vi "ZDataVIS_LineCuts.vi"(4 "Intensity Plot":refnum<vi>, 6 "e^2/h?":bool, 7 "tpose":bool, 8 "error in (no error)":errorcluster, 9 "Decimated X values":dbl[](array[numeric]), 10 "Arr of Y arrays (intensity info)":dbl[][](array[numeric]), 11 "State Wire IN":T1={"Core"={"Current VI Reference"=refnum, "Close Panel on Exit?"=FALSE}, "Sweep Data Cluster"={"Vfast"=[], "Vslow"=[], "Vslowest"=[], "Comments"="", "Scan names"=[]}, "Cursor Info"={"Fast Index"=[], "Slow Index"=0.0, "Slow Indices"=[], "Raw Cursor Position"={"X"=0.0, "Y"=0.0}, "Field / temp"=0}, "Scan names"=[], "Data DVR"=refnum, "Arr of Y arrays (intensity info)"=[], "Decimated X values"=[], "X Step Info"={"X Low"=-0.1, "X High"=0.1, "X Step"=4e-05}, "Voffset -2T"=0.0} {"X Step Info"."X Step" format="%#_6p"; "X Step Info"."X High" format="%#_6p"; "X Step Info"."X Low" format="%#_6p"}) -> (0 "error out":errorcluster, 1 "X line cut":cluster{dbl[], dbl[]}(graph), 2 "Y line cut":cluster{"Vfast":dbl[], dbl[]}(graph), 3 "State Wire OUT":T1={"Core"={"Current VI Reference"=refnum, "Close Panel on Exit?"=FALSE}, "Sweep Data Cluster"={"Vfast"=[], "Vslow"=[], "Vslowest"=[], "Comments"="", "Scan names"=[]}, "Cursor Info"={"Fast Index"=[], "Slow Index"=0.0, "Slow Indices"=[], "Raw Cursor Position"={"X"=0.0, "Y"=0.0}, "Field / temp"=0}, "Scan names"=[], "Data DVR"=refnum, "Arr of Y arrays (intensity info)"=[], "Decimated X values"=[], "X Step Info"={"X Low"=-0.1, "X High"=0.1, "X Step"=4e-05}, "Voffset -2T"=0.0} {"X Step Info"."X Step" format="%#_6p"; "X Step Info"."X High" format="%#_6p"; "X Step Info"."X Low" format="%#_6p"})   [LabVIEW 2016]
uses:
  ZDataVIS_StateWire.ctl
  <vilib>/Utility/miscctls.llb/LVPointDoubleTypeDef.ctl
panel:
  out "s":i32
  out "Sweep Data Cluster.Vfast":dbl[][](array[numeric])
  # "cursor x"
  # "cursor y"
  # "cursor x"
  # "cursor y"
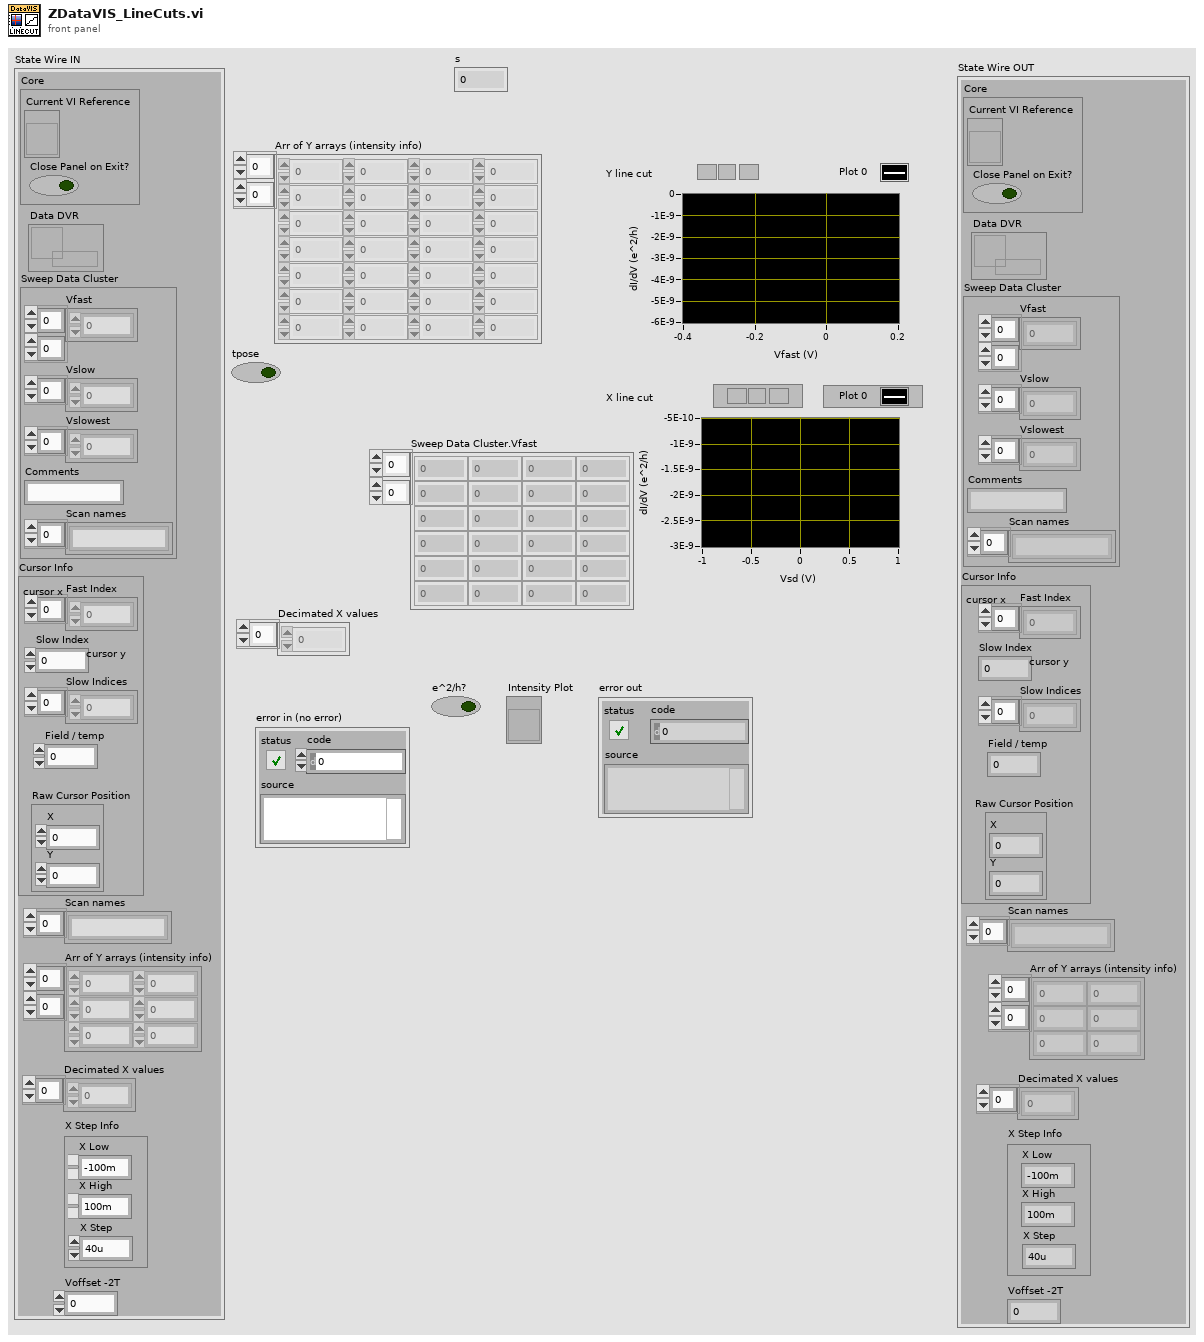
[diagram p1: front panel]
types:
  T1 = typedef "ZDataVIS_StateWire.ctl" = cluster{"Core":cluster{"Current VI Reference":refnum<vi>, "Close Panel on Exit?":bool}, "Sweep Data Cluster":cluster{"Vfast":dbl[][], "Vslow":dbl[], "Vslowest":dbl[], "Comments":string, "Scan names":string[]}, "Cursor Info":cluster{"Fast Index":dbl[], "Slow Index":dbl, "Slow Indices":dbl[], "Raw Cursor Position":T2, "Field / temp":i32}, "Scan names":string[], "Data DVR":refnum<data-value>, "Arr of Y arrays (intensity info)":dbl[][], "Decimated X values":dbl[], "X Step Info":cluster{"X Low":dbl, "X High":dbl, "X Step":dbl}, "Voffset -2T":dbl}
  T2 = typedef "LVPointDoubleTypeDef.ctl" = cluster{"X":dbl, "Y":dbl}
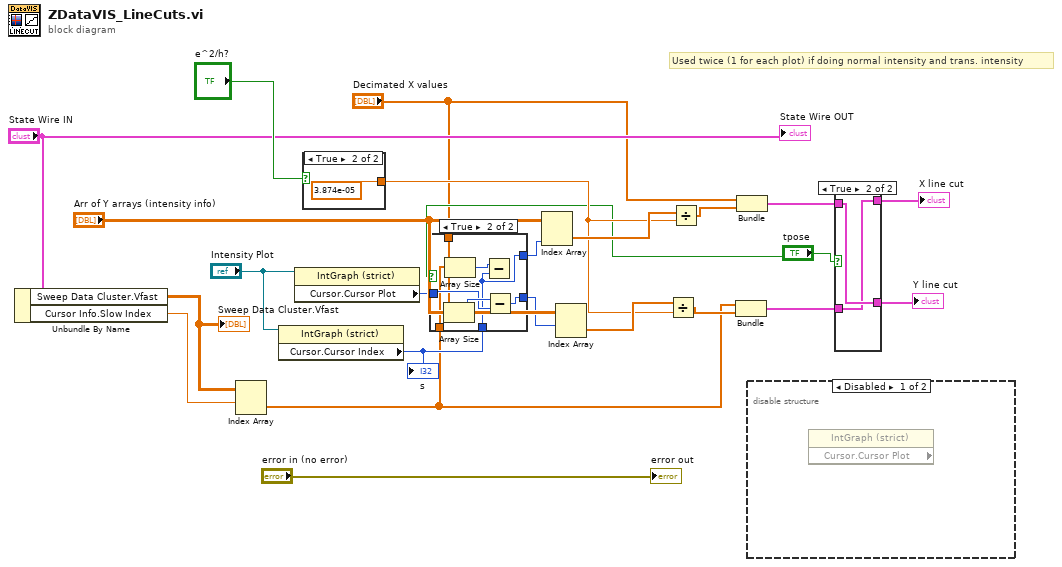
[diagram p0: block diagram]
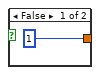
[diagram p5: hidden frame]
diagram:
  # "Used twice (1 for each plot) if doing normal intensity and trans. intensity"
  n1 = Unbundle By Name("State Wire IN") -> ("Sweep Data Cluster.Vfast"=w15:dbl[][], "Cursor Info.Slow Index"=w14:dbl)
  "Sweep Data Cluster.Vfast" <- w15
  n2 = Index Array(array=w15, index (row)=w14) -> (element=w2:dbl[])  [unwired: 1 in]
  n3 = property on="Property Node" class="IntGraph (strict)"(reference="Intensity Plot") -> ("Cursor.Cursor Index"=w5:i32)  [unwired: 1 in, 2 out]
  "s" <- w5
  n4 = property on="Property Node" class="IntGraph (strict)"(reference="Intensity Plot") -> ("Cursor.Cursor Plot"=w4:i32)  [unwired: 1 in, 2 out]
  n5 = case shown="True" "e^2/h?" {
    tunnel: [1 3.874e-05] -> w18
    frame False {
    }
    frame True {
    }
  }
  n6 = case shown="True" "tpose" {
    tunnel: [w27 w28] -> w7
    tunnel: [w26 w33] -> w6
    tunnel: w5 -> [w26 w28]
    tunnel: w4 -> [w27 w31]
    tunnel: w2 -> [_ w30]
    tunnel: "Decimated X values" -> [_ w29]
    frame False {
    }
    frame True {
      n7 = Array Size(array=w29) -> (size(s)=w32:i32)
      n8 = Array Size(array=w30) -> (size(s)=w34:i32)
      n9 = Subtract(x=w34, y=w28) -> ()  [unwired: 1 out]
      n10 = Subtract(x=w32, y=w31) -> (x-y=w33:i32)
    }
  }
  n11 = Index Array(array="Arr of Y arrays (intensity info)", index (col)=w7) -> (element=w20:dbl[])  [unwired: 1 in]
  n12 = Index Array(array="Arr of Y arrays (intensity info)", index (row)=w6) -> (element=w19:dbl[])  [unwired: 1 in]
  n13 = Divide(x=w19, y=w18) -> (x/y=w17:dbl[])
  n14 = Divide(x=w20, y=w18) -> (x/y=w22:dbl[])
  n15 = Bundle("Vfast"=w2, w17) -> (w8:cluster{"Vfast":dbl[], dbl[]})  [unwired: 1 in]
  n16 = Bundle("Decimated X values"="Decimated X values", w22) -> (w10:cluster{"Decimated X values":dbl[], dbl[]})  [unwired: 1 in]
  n17 = disable-structure shown="Disabled" {
    frame Disabled {
      n18 = property on="Property Node" class="IntGraph (strict)" props=["Cursor", "Cursor Plot"]() -> ()  [unwired: 2 in, 3 out]
    }
    frame Enabled {
    }
  }
  n19 = case shown="True" "tpose" {
    tunnel: [w35 w38] -> w11
    tunnel: w10 -> [w36 w38]
    tunnel: [w36 w37] -> w9
    tunnel: w8 -> [w35 w37]
    frame False {
    }
    frame True {
    }
  }
  "Y line cut" <- w11
  "X line cut" <- w9
  "error out" <- "error in (no error)"
  "State Wire OUT" <- "State Wire IN"
